vi "Update UI.vi"(8 "error in (no error)":errorcluster, 10 "Status":string, 11 "Execution UI In":refnum<class "Execution UI.lvclass">) -> (0 "error out":errorcluster, 3 "Execution UI Out":refnum<class "Execution UI.lvclass">)   [LabVIEW 2020, in "Execution UI.lvclass"]
uses:
  Execution UI.lvclass
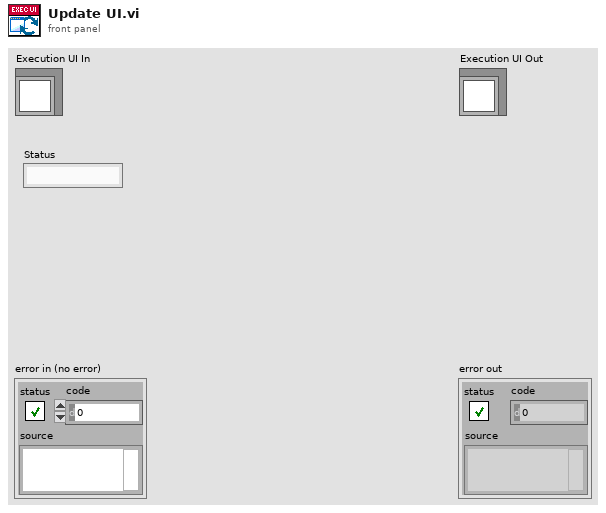
[diagram p1: front panel]
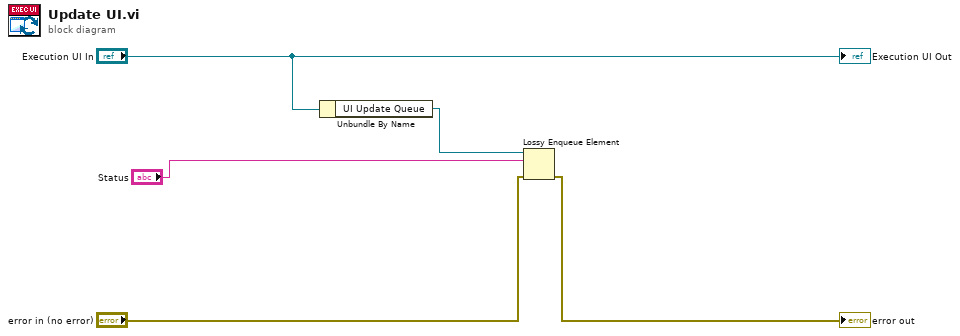
[diagram p0: block diagram]
diagram:
  n1 = Unbundle By Name("Execution UI In") -> ("UI Update Queue"=w4:refnum<queue>)
  n2 = Lossy Enqueue Element(queue=w4, element="Status", error in (no error)="error in (no error)") -> (error out=→"error out":errorcluster)  [unwired: 3 out]
  "Execution UI Out" <- "Execution UI In"
